vi "PH_4_Pos_Selector.constructor.vi"(0 "name":string, 2 "data in":string, 5 "error in(no error)":errorcluster) -> (14 "i ref out":refnum<vi>, 16 "data out":string, 19 "error out":errorcluster)   [LabVIEW 2014, in "PH_4_Pos_Selector.lvlib"]
doc: "This class is forseen to control up to two Sixpack Axes (classes: Trinamic_Axis and Trinamic_Controller).\n\nThis class is part of the PHELIX user layer.\n\nauthor: Stefan Götte, GSI\n\nLicense Agreement for this software:\n\nCopyright (C)\nGesellschaft für Schwerionenforschung, GSI\nPlanckstr. 1\n64291 Darmstadt\nGermany\n\nContact: D.Beck@gsi.de \n\nThis program is free software; you can redistribute it and/or modify it under the terms of the \nGNU General Public License as published by the Free Software Foundation; either version 2 of \nthe license, or (at your option) any later version.\n\nThis program is distributed in the hope that it will be useful, but WITHOUT ANY WARRANTY; \nwithout even the implied warranty of MERCHANTABILITY or FITNESS FOR A PARTICULAR PURPOSE. See the GNU General License for more details (http://www.gnu.org).\n\nGesellschaft für Schwerionenforschung, GSI\nPlanckstr. 1, 64291 Darmstadt, Germany\nFor all questions and ideas contact: M.Richter@gsi.de, H.Brand@gsi.de or D.Beck@gsi.de.\nLast update: 16-JUN-2004"
uses:
  PH_4_Pos_Selector.lvlib
  PH_AxisGUI_6P/PH_AxisGUI_6P.lvlib
  CS_Core/CSObj/CSObj.lvlib
  PH_Basics/PH_Class/PH_Class.lvlib
  PH_Basics/PH_PSDBWriter/PH_PSDBWriter.lvlib
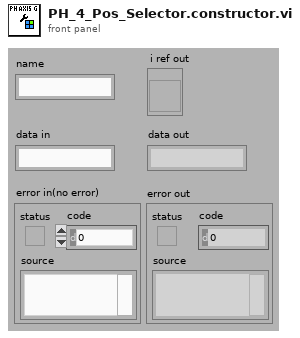
[diagram p1: front panel]
types:
  T1 = enum16{"SetAttribute", "GetAttribute", "CreateAttribute", "DestroyAttribute", "DestroyAllAtributes"}
  T2 = typedef "PH_4_Pos_Selector.lvlib/PH_4_Pos_Selector.Position Selector.ctl" = u16
  T3 = typedef "PH_4_Pos_Selector.lvlib/PH_4_Pos_Selector.i attribute.ctl" = cluster{"GUI Refs":cluster{"Position I":refnum<vi>, "Position II":refnum<vi>, "Position III":refnum<vi>, "Position IV":refnum<vi>, "rel. Mode?":refnum<vi>, "Define Selector":refnum<vi>}, "Current Position":T2, "Service ID Position":i32, "Position Array":T4[], "Description Array":string[], "relative Mode":bool, "Wanted Define Selector Position":string}
  T4 = typedef "PH_4_Pos_Selector.lvlib/PH_4_Pos_Selector.Position.ctl" = cluster{"Axis 1":dbl, "Axis 2":dbl}
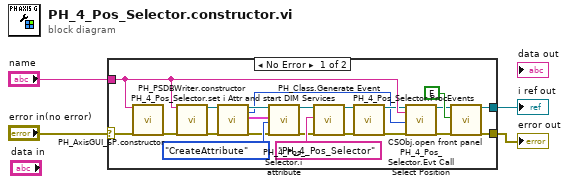
[diagram p0: block diagram]
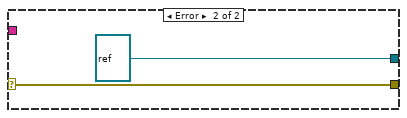
[diagram p2: hidden frame]
diagram:
  n1 = case shown="No Error" "error in(no error)" {
    selector: "error in(no error)" -> [w22 w28]
    tunnel: [w24 w28] -> w4
    tunnel: [w23 refnum<vi> refnum ("i ref out")] -> w3
    tunnel: "name" -> [w25 _]
    frame No Error {
      n2 = call "PH_AxisGUI_6P.constructor.vi"("name"=w25, "error in(no error)"=w22) -> ("error out"=w13:errorcluster)  [unwired: 15 in, 2 out]
      n3 = call "PH_PSDBWriter.constructor.vi"("name"=w25, "error in"=w13) -> ("i ref out"=w11:refnum<vi>, "error out"=w12:errorcluster)  [unwired: 15 in, 1 out]
      n4 = call "PH_4_Pos_Selector.set i Attr and start DIM Services.vi"("i ref in"=w11, "error in (no error)"=w12) -> ("i ref out"=w10:refnum<vi>, "Wanted start position"=w5:T2, "i Attr"=w9:T3, "error out"=w8:errorcluster)  [unwired: 14 in]
      n5 = call "PH_4_Pos_Selector.i attribute.vi"("VI Refnum"=w10, "CLASS.i attribute"=w9, "Action"=T1."CreateAttribute", "error in (no error)"=w8) -> ("VI Refnum out"=w14:refnum<vi>, "error out"=w17:errorcluster)  [unwired: 13 in, 1 out]
      n6 = call "PH_Class.Generate Event.vi"("i ref in"=w14, "Class"="PH_4_Pos_Selector", "error in (no error)"=w17) -> ("i ref out"=w15:refnum<vi>, "error out"=w16:errorcluster)  [unwired: 15 in]
      n7 = call "PH_4_Pos_Selector.ProcEvents.vi"("i ref in"=w15, "error in"=w16) -> ("i ref out"=w6:refnum<vi>, "error out"=w7:errorcluster)  [unwired: 16 in]
      n8 = call "PH_4_Pos_Selector.Evt Call Select Position.vi"("i ref in"=w6, "4 Pos instance"=w25, "Wanted Position"=w5, "error in"=w7) -> ("i ref out"=w19:refnum<vi>, "error out"=w18:errorcluster)  [unwired: 14 in]
      n9 = call "CSObj.open front panel.vi"("i ref in"=w19, "frontPanelOpen"=FALSE ("front panel open"), "error in (no error)"=w18) -> ("i ref out"=w23:refnum<vi>, "error out"=w24:errorcluster)  [unwired: 15 in]
    }
    frame Error {
    }
  }
  "i ref out" <- w3
  "error out" <- w4
